vi "Init Order Queue.vi"(8 "error in (no error)":errorcluster, 11 "Agent in":refnum<class "Agent.lvclass">) -> (0 "error out":errorcluster, 1 "created new?":bool, 3 "Agent out":refnum<class "Agent.lvclass">)   [LabVIEW 2019, in "Agent.lvclass"]
doc: "Create the order queue the agent uses to keep track of orders waiting to be processed"
uses:
  Agent.lvclass
  Order/Order.lvclass
  Agent.lvclass/Agent.ctl
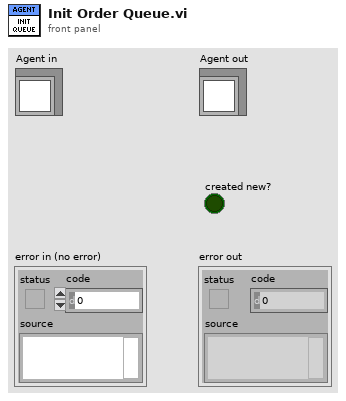
[diagram p1: front panel]
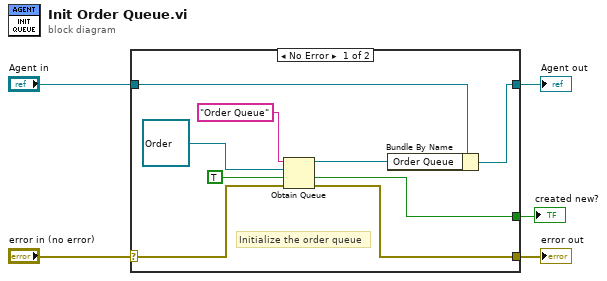
[diagram p0: block diagram]
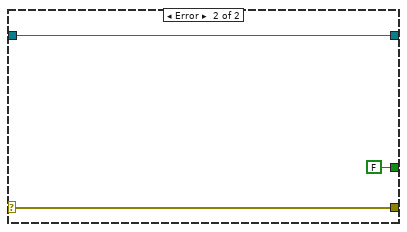
[diagram p2: hidden frame]
diagram:
  n1 = case shown="No Error" "error in (no error)" {
    selector: "error in (no error)" -> [w9 w16]
    tunnel: [w8 w16] -> w4
    tunnel: [w13 w17] -> w2
    tunnel: "Agent in" -> [w14 w17]
    tunnel: [w6 FALSE ("created new?")] -> w1
    frame No Error {
      # "Initialize the order queue"
      n2 = Obtain Queue(name (unnamed)="Order Queue", element data type=refnum<class "Order.lvclass"> refnum ("Order.lvclass"), create if not found? (T)=TRUE, error in (no error)=w9) -> (queue out=w7:refnum<queue>, created new?=w6:bool, error out=w8:errorcluster)  [unwired: 1 in]
      n3 = Bundle By Name(cluster=w14, "Order Queue"=w7) -> (w13:refnum<class "Agent.lvclass">)
    }
    frame Error {
    }
  }
  "error out" <- w4
  "Agent out" <- w2
  "created new?" <- w1
